vi "reset_TRIG2.vi"(8 "error in (no error)":errorcluster, 11 "VISA resource name":refnum<visa-resource-name>) -> (0 "error out":errorcluster, 3 "VISA resource name out":refnum<visa-resource-name>)   [LabVIEW 2012]
doc: "This vi resets TRIG2 (DG645) to its defaultsetup and then configures a default setup for the chirped pulse setup.\nThis includes activating the burst mode (3 bursts, 100us burst period), setting polarities as well as setting all delays and durations to 0."
uses:
  global.vi
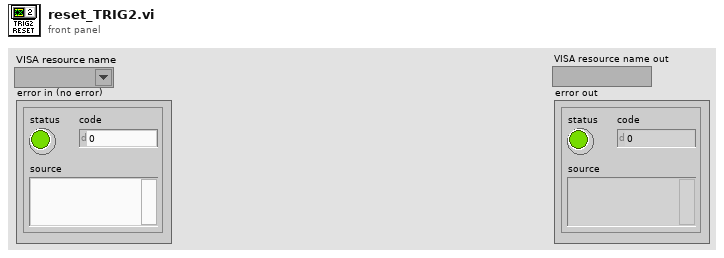
[diagram p1: front panel]
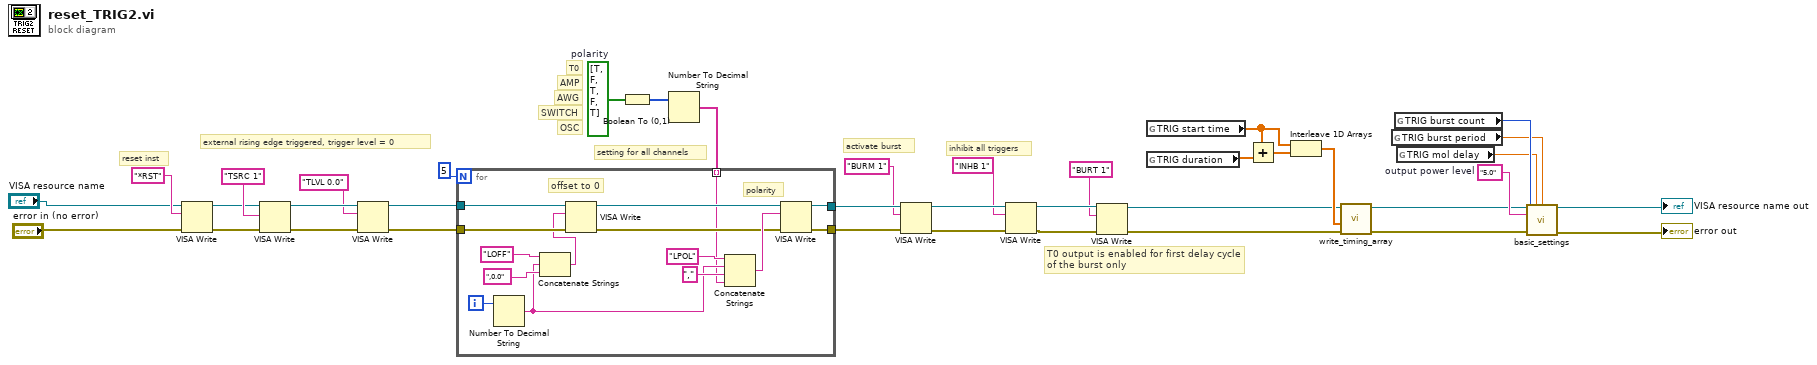
[diagram p0: block diagram]
diagram:
  w12 = "5.0"  # output power level
  w29 = bool[] [TRUE, FALSE, TRUE, FALSE, TRUE]  # polarity
  # "T0 output is enabled for first delay cycle \nof the burst only"
  # "inhibit all triggers"
  # "activate burst"
  # "OSC"
  # "SWITCH"
  # "AWG"
  # "AMP"
  # "T0"
  # "reset inst"
  # "setting for all channels"
  # "external rising edge triggered, trigger level = 0"
  n1 = VISA Write(VISA resource name="VISA resource name", write buffer="*RST", error in (no error)="error in (no error)") -> (VISA resource name out=w34:refnum<visa-resource-name>, error out=w35:errorcluster)  [unwired: 1 out]
  n2 = VISA Write(VISA resource name=w34, write buffer="TSRC 1" ("Query 2"), error in (no error)=w35) -> (VISA resource name out=w26:refnum<visa-resource-name>, error out=w36:errorcluster)  [unwired: 1 out]
  n3 = VISA Write(VISA resource name=w26, write buffer="TLVL 0.0", error in (no error)=w36) -> (VISA resource name out=w25:refnum<visa-resource-name>, error out=w27:errorcluster)  [unwired: 1 out]
  n4 = Boolean To (0,1)(Boolean=w29) -> (0, 1=w30:i16[])
  n5 = Number To Decimal String(number=w30) -> (decimal integer string=w28:string[])  [unwired: 1 in]
  n6 = for {
    N: 5 -> [_]
    tunnel: w25 -> [w51]
    tunnel: [w42] -> w21
    tunnel: w27 -> [w50]
    tunnel: [w41] -> w23
    tunnel: w28 -> [w39] mode=indexing
    i -> [w49]
    # "polarity"
    # "offset to 0"
    n7 = Number To Decimal String(number=w49) -> (decimal integer string=w40:string)  [unwired: 1 in]
    n8 = Concatenate Strings("LOFF" ("Query 2"), w40, ",0.0" ("Query 2")) -> (w46:string)
    n9 = VISA Write(VISA resource name=w51, write buffer=w46, error in (no error)=w50) -> (VISA resource name out=w42:refnum<visa-resource-name>, error out=w41:errorcluster)  [unwired: 1 out]
    n10 = Concatenate Strings("LPOL" ("Query 2"), w40, "," ("string"), w39) -> (w44:string)
    n11 = VISA Write(VISA resource name=w42, write buffer=w44, error in (no error)=w41) -> ()  [unwired: 3 out]
  }
  n12 = VISA Write(VISA resource name=w21, write buffer="BURM 1", error in (no error)=w23) -> (VISA resource name out=w18:refnum<visa-resource-name>, error out=w22:errorcluster)  [unwired: 1 out]
  n13 = VISA Write(VISA resource name=w18, write buffer="INHB 1", error in (no error)=w22) -> (VISA resource name out=w16:refnum<visa-resource-name>, error out=w19:errorcluster)  [unwired: 1 out]
  n14 = VISA Write(VISA resource name=w16, write buffer="BURT 1", error in (no error)=w19) -> (VISA resource name out=w5:refnum<visa-resource-name>, error out=w4:errorcluster)  [unwired: 1 out]
  n15 = global read "global.vi" "TRIG start time"() -> (w9:dbl[])
  n16 = global read "global.vi" "TRIG duration"() -> (w10:dbl[])
  n17 = Add(x=w9, y=w10) -> (x+y=w8:dbl[])
  n18 = Interleave 1D Arrays(w9, w8) -> (w11:dbl[])
  n19 = call "write_timing_array.vi"("error in"=w4, "delay array"=w11, "VISA resource in"=w5) -> ("error out 2"=w6:errorcluster, "VISA resource out"=w7:refnum<visa-resource-name>)  [unwired: 3 in]
  n20 = global read "global.vi" "TRIG burst period"() -> (w13:dbl)
  n21 = global read "global.vi" "TRIG burst count"() -> (w14:i32)
  n22 = global read "global.vi" "TRIG mol delay"() -> (w1:dbl)
  n23 = call "basic_settings.vi"("VISA resource name"=w7, "molecular delay"=w1, "burst period (s)"=w13, "burst count"=w14, "power level"=w12, "error in (no error)"=w6) -> ("VISA resource name out"=→"VISA resource name out":refnum<visa-resource-name>, "error out"=→"error out":errorcluster)  [unwired: 8 in]
